vi "Get Spectrum.vi"(0 "Filter in":refnum<class "Filter.lvclass">, 7 "Npts":i32, 11 "error in (no error)":errorcluster) -> (4 "Filter out":refnum<class "Filter.lvclass">, 8 "spectrum":cdb[](array[numeric]), 15 "error out":errorcluster)   [LabVIEW 2020, in "Filter.lvclass"]
uses:
  Filter.lvclass
  Filter.lvclass/Filter.ctl
  <vilib>/Analysis/2dsp.llb/Real FFT.vi
  <vilib>/Analysis/NI_AALBase.lvlib
  <vilib>/Analysis/NI_AALPro.lvlib
panel:
  out "r":dbl[](array[numeric])
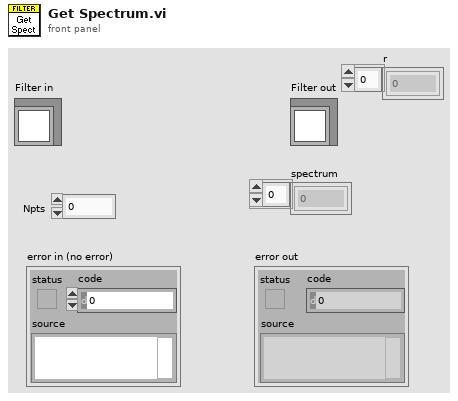
[diagram p1: front panel]
types:
  T1 = enum16{"Lowpass", "Highpass", "Bandpass", "Bandstop", "OFF"}
  T2 = typedef "Filter.lvclass/Shape.ctl" = enum16{"OFF", "Lowpass", "Highpass", "Bandpass", "Bandstop"}
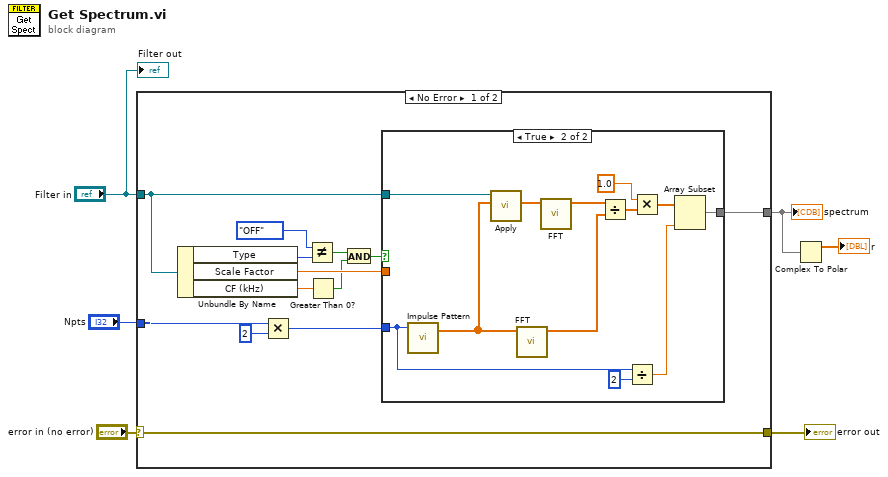
[diagram p0: block diagram]
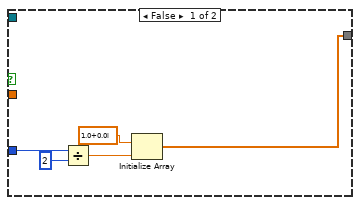
[diagram p2: hidden frame]
diagram:
  n1 = case shown="No Error" "error in (no error)" {
    selector: "error in (no error)" -> [w18 w37]
    tunnel: "Filter in" -> [w10 _]
    tunnel: "Npts" -> [w14 _]
    tunnel: [w19 _] -> w2
    tunnel: [w18 w37] -> w4
    frame No Error {
      n2 = Unbundle By Name(w10) -> ("Type"=w13:T2, "Scale Factor"=w17:dbl, "CF (kHz)"=w8:dbl)
      n3 = Multiply(x=w14, y=2) -> (x*y=w16:i32)
      n4 = Not Equal?(x=T1."OFF", y=w13) -> (x != y?=w11:bool)
      n5 = Greater Than 0?(x=w8) -> (x > 0?=w7:bool)
      n6 = And(x=w11, y=w7) -> (x .and. y?=w9:bool)
      n7 = case shown="True" w9 {
        tunnel: w16 -> [w23 w28]
        tunnel: [w20 w31] -> w19
        tunnel: w17 -> [_ _]
        tunnel: w10 -> [_ w25]
        frame False {
          n8 = Divide(x=w23, y=2) -> (x/y=w22:dbl)
          n9 = Initialize Array(cdb 1.0+0.0i ("element"), w22) -> (w20:cdb[])
        }
        frame True {
          n10 = call <vilib>:"Impulse Pattern.vi"("samples"=w28) -> ("Impulse Pattern"=w27:dbl[])  [unwired: 2 in, 1 out]
          n11 = call "Apply.vi"("Array in"=w27, "Filter in"=w25) -> ("Array out"=w29:dbl[])  [unwired: 7 in, 2 out]
          n12 = call-poly <vilib>:"FFT.vi"("X"=w27) -> ("FFT {X}"=w35:cdb[])  [unwired: 9 in, 1 out]
          n13 = call-poly <vilib>:"FFT.vi"("X"=w29) -> ("FFT {X}"=w36:cdb[])  [unwired: 9 in, 1 out]
          n14 = Divide(x=w36, y=w35) -> (x/y=w34:cdb[])
          n15 = Divide(x=w28, y=2) -> (x/y=w32:dbl)
          n16 = Multiply(x=1.0 ("Scale Factor"), y=w34) -> (x*y=w30:cdb[])
          n17 = Array Subset(array=w30, length=w32) -> (w31:cdb[])  [unwired: 1 in]
        }
      }
    }
    frame Error {
    }
  }
  "error out" <- w4
  "spectrum" <- w2
  n18 = Complex To Polar(r * e^(i*theta)=w2) -> (r=→"r":dbl[])  [unwired: 1 out]
  "Filter out" <- "Filter in"
